vi "Won Game User Prompt and State Transition Out.vi"(8 "error in (no error)":errorcluster, 11 "Player 1 wins":bool) -> (0 "error out":errorcluster, 2 "Next State - Out":T1, 3 "String - Out":string)   [LabVIEW 2021]
uses:
  Controls/State.ctl
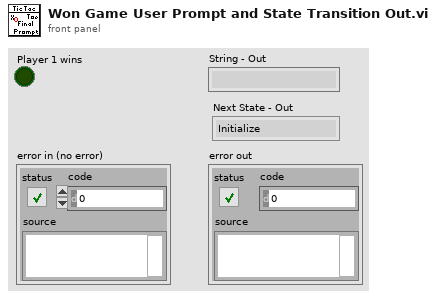
[diagram p1: front panel]
types:
  T1 = typedef "State.ctl" = enum16{"Initialize", "Wait for Event", "Set Left Upp", "Set Left Mid", "Set Left Bot", "Set Middle Upp", "Set Middle Mid", "Set Middle Bot", "Set Right Upp", "Set Right Mid", "Set Right Bot", "Check Game Status", "Exit"}
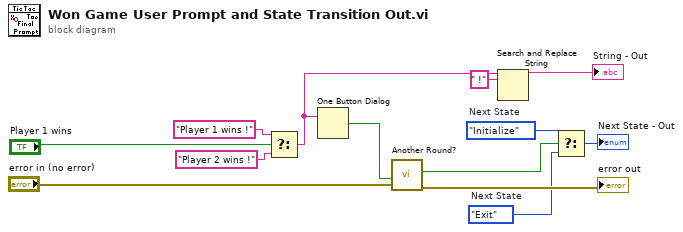
[diagram p0: block diagram]
diagram:
  w11 = State."Exit"  # Next State
  w10 = State."Initialize"  # Next State
  n1 = Select(t="Player 1 wins !" ("O Const"), s="Player 1 wins", f="Player 2 wins !" ("O Const")) -> (s? t:f=w4:string)
  n2 = One Button Dialog(message=w4) -> (true=w1:bool)  [unwired: 1 in]
  n3 = call "Another Round?"("error in (no error)"="error in (no error)", "Enable"=w1) -> ("error out"=→"error out":errorcluster, "Yes"=w9:bool)  [unwired: 8 in]
  n4 = Search and Replace String(input string=w4, search string=" !") -> (result string=→"String - Out":string)  [unwired: 6 in, 3 out]
  n5 = Select(t=w10, s=w9, f=w11) -> (s? t:f=→"Next State - Out":T1)
